vi "PreviewInstall.vi"(8 "Error In":errorcluster, 9 "Include Recommended?":bool, 10 "Version":string, 11 "Package Name":string) -> (0 "Error Out":errorcluster, 2 "Install Command":string, 3 "Preview":string)   [LabVIEW 2019, in "CEPM.lvlib"]
uses:
  CEPM.lvlib
  <vilib>/Utility/sysdir.llb/System Directory Type.ctl
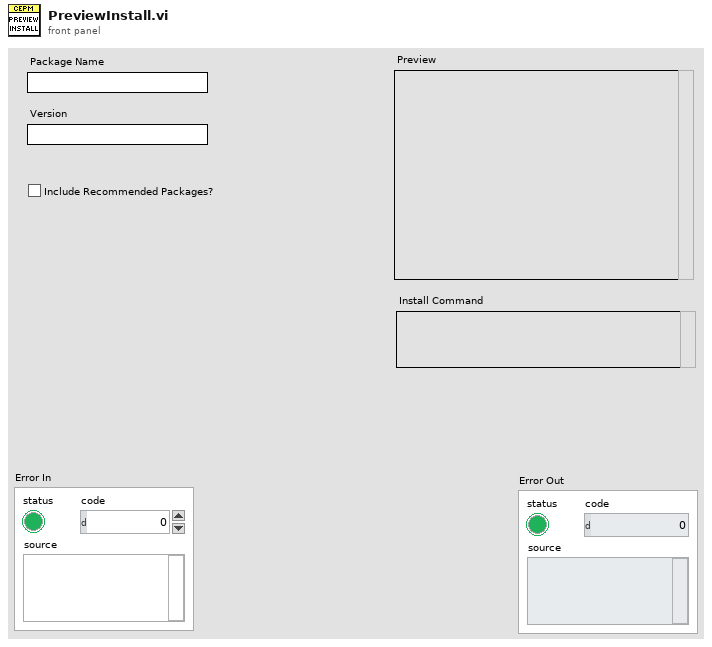
[diagram p1: front panel]
types:
  T1 = typedef "System Directory Type.ctl" = i32
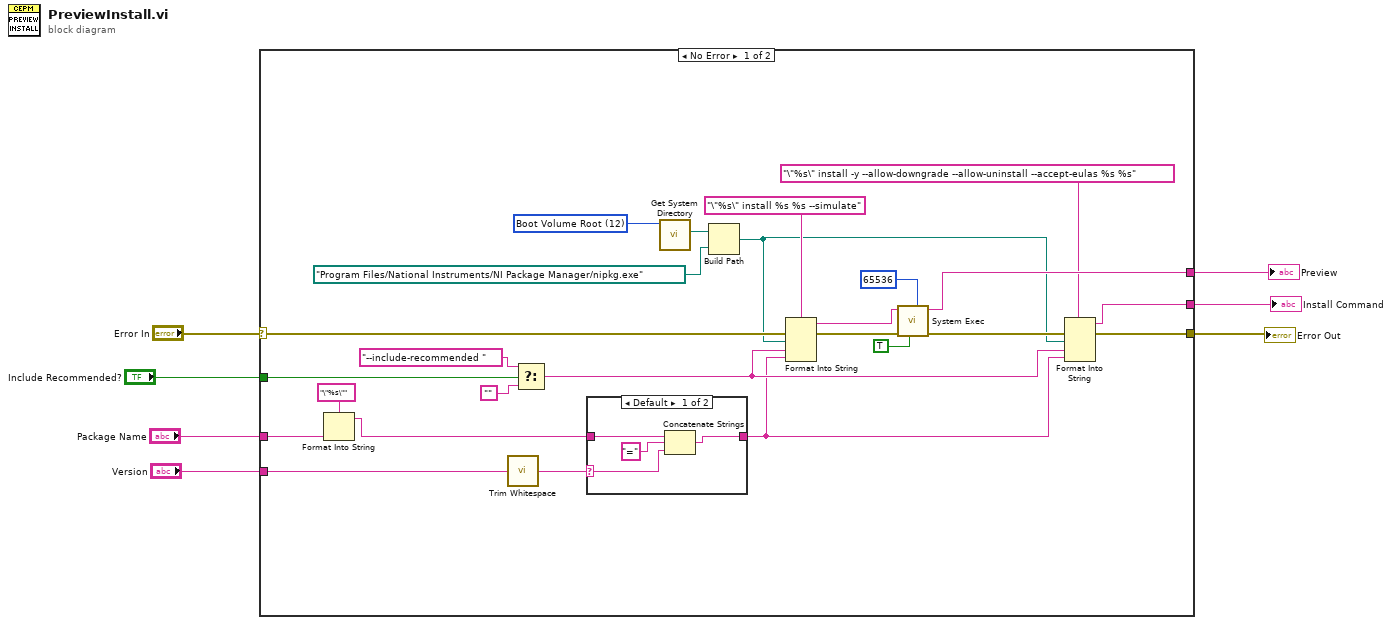
[diagram p0: block diagram]
diagram:
  n1 = case shown="No Error" "Error In" {
    selector: "Error In" -> [w32 w38]
    tunnel: [w16 w38] -> w6
    tunnel: "Version" -> [w26 _]
    tunnel: "Package Name" -> [w10 _]
    tunnel: [w22 _] -> w3
    tunnel: "Include Recommended?" -> [w19 _]
    tunnel: [w11 _] -> w1
    frame No Error {
      w28 = T1 12 items=["User Home"=0, "User Desktop"=1, "User Documents"=2, "User Application Data"=3, "User Preferences"=4, "User Temporary"=5, "Public Documents"=6, "Public Application Data"=7, "Public Preferences"=8, "Public Cache"=13, "System Core Libraries"=9, "System Installed Libraries"=10, "Application Files"=11, "Boot Volume Root"=12] ("system directory type")
      n2 = Format Into String(format string="\"%s\"", w10) -> (resulting string=w8:string)  [unwired: 2 in, 1 out]
      n3 = call <vilib>:"Trim Whitespace.vi"("string"=w26) -> ("trimmed string"=w18:string)  [unwired: 1 in]
      n4 = Select(t="--include-recommended ", s=w19, f="") -> (s? t:f=w14:string)
      n5 = case shown="Default" w18 {
        selector: w18 -> [w35 _]
        tunnel: w8 -> [w36 w37]
        tunnel: [w33 w37] -> w13
        frame Default {
          n6 = Concatenate Strings(w36, "=" ("string"), w35) -> (w33:string)
        }
        frame "" {
        }
      }
      n7 = call <vilib>:"Get System Directory.vi"("system directory type"=w28) -> ("system directory"=w29:path)  [unwired: 10 in]
      n8 = Build Path(base path=w29, name or relative path=path "Program Files/National Instruments/NI Package Manager/nipkg.exe" ("working directory")) -> (appended path=w15:path)
      n9 = Format Into String(format string="\"%s\" install %s %s --simulate", error in=w32, w15, w14, w13) -> (resulting string=w25:string, error out=w31:errorcluster)  [unwired: 1 in]
      n10 = call <vilib>:"System Exec.vi"("expected output size  (4096)"=u32 65536, "run minimized? (F)"=TRUE, "error in (no error)"=w31, "command line"=w25) -> ("error out"=w17:errorcluster, "standard output"=w22:string)  [unwired: 4 in, 2 out]
      n11 = Format Into String(format string="\"%s\" install -y --allow-downgrade --allow-uninstall --accept-eulas %s %s", error in=w17, w15, w14, w13) -> (resulting string=w11:string, error out=w16:errorcluster)  [unwired: 1 in]
    }
    frame Error {
    }
  }
  "Error Out" <- w6
  "Preview" <- w3
  "Install Command" <- w1
